vi "SiPM_Oscilloscope_tests.vi"(1 "Results Directory":path=path "C:/Users/johnk/Desktop/ESA_Scintillator_Data", 2 "Isotope":string) -> ()   [LabVIEW 2015]
doc: "This example shows how to configure multiple channels and acquire waveforms from multiple channels."
uses:
  <instrlib>/RIGOL DP800 Series/Public/Channels.ctl
  Agilent_lib/Public/Data/Read Measurement (Current Value).vi
  Agilent_lib/Public/Configure/Trigger/Configure Trigger (Edge).vi
  Agilent_lib/Agilent 2000 3000 X-Series.lvlib
  <vilib>/Analysis/NI_AALPro.lvlib
  <vilib>/Analysis/NI_AALBase.lvlib
  <instrlib>/RIGOL DG4000 Series/RIGOL DG4000 Series.lvlib
  <instrlib>/RIGOL DP800 Series/RIGOL DP800 Series.lvlib
panel:
  in  "x = y?":bool
  in  "Enable\nVernier":bool
  in  "Enable \nREF \nBNC":bool
  in  "Time Base Type":i32(ring) items=["Main", "Window", "XY", "Roll"]
  out "appended array":i32[](array[numeric])
  in  "Tab Control":enum32{"Page 2"}(tab)
  in  "Set Manual Temp?":bool
  in  "Temperature":string
  in  "Settings Button":bool
  in  "Stop Button":bool
  in  "Free Run":bool
  in  "Range":dbl(slide)=0.001 min=2e-08 max=500.0 scale=0.0..0.001
  in  "Pulse Width (s)":ext=1.25e-8 format="%#.3p"
  in  "Read DC":bool
  in  "Out Enable 2":bool
  in  "Set DC":bool
  out "Actual V Level  2":dbl caption="Actual Level (V)" format="%#.3g"
  out "Actual Level (A)":dbl caption="Actual Current Level" format="%#.3g"
  in  "VISA resource name":refnum<visa-resource-name>="USB0::0x0957::0x1780::MY56270584::INSTR"
  out "BIAS Voltage":dbl
  in  "Read Temperature":bool
  out "Celcius":dbl(slide) scale=0.0..30.0
  in  "Trigger Source":i32(ring) items=["Channel 1"=0, "Channel 2"=1, "Channel 3"=2, "Channel 4"=3, "D0"=13, "D1"=14, "D2"=15, "D3"=16, "D4"=17, "D5"=18, "D6"=19, "D7"=20, "D8"=21, "D9"=22, "D10"=23, "D11"=24, "D12"=25, "D13"=26, "D14"=27, "D15"=28, "External"=29, "Power Line"=30, "Waveform Generator"=31]
  in  "Input \nCoupling":i32(ring)=1 items=["AC Coupling", "DC Coupling", "Low Frequency Reject"]
  in  "Edge \nSlope":i32(ring) items=["Pos", "Neg", "Either", "Alt"]
  in  "Trigger Level (V)":dbl(knob)=0.02 min=-10.0 max=10.0 step=0.01 scale=0.0..5.0
  out "HV Indicator":bool
  in  "EN 4":bool
  in  "Ch 4 Vertical Scale":dbl(knob)=5.0 min=0.0 max=5.0 step=0.05 scale=0.0..5.0
  in  "CH 4  offset":dbl(knob) min=-10.0 max=10.0 step=0.01 scale=0.0..10.0
  in  "Ch3 Vertical Scale":dbl(knob)=5.0 min=0.0 max=5.0 step=0.05 scale=0.0..5.0
  in  "CH 3  offset":dbl(knob) min=-10.0 max=10.0 step=0.01 scale=0.0..10.0
  in  "EN 3":bool
  in  "EN 2":bool=TRUE
  in  "Ch 2 Vertical Scale":dbl(knob)=0.05 min=0.0 max=5.0 step=0.05 scale=0.0..5.0
  in  "CH 2  offset":dbl(knob)=0.18 min=-10.0 max=10.0 step=0.01 scale=0.0..10.0
  in  "Ch1 Vertical Scale":dbl(knob)=0.05 min=0.0 max=5.0 step=0.001 scale=0.0..5.0
  in  "CH 1  offset":dbl(knob)=0.18 min=-10.0 max=10.0 step=0.01 scale=0.0..10.0
  in  "EN":bool=TRUE
  out "Oscilloscope Waveform":waveform(dbl)[](graph)
  in  "Impedance":i32(ring)=1 items=["1 MOhm", "50 Ohm"]
  in  "Coupling":i32(ring)=1 items=["AC", "DC"]
  in  "Vertical Setting":i32(ring) items=["Vertical Scale", "Vertical Range"]
  in  "Vertical Range":dbl=40.0
  in  "Time per Division":dbl(knob)=2e-07 scale=0.0..1.0
  in  "Horizontal \nPosition":dbl(knob) scale=0.0..1.0
  in  "Ch1":u8=1 min=1 max=10 step=9
  in  "Ch2":u8=1 min=1 max=10 step=9
  in  "Ch3":u8=10 min=1 max=10 step=9
  in  "Ch4":u8=10 min=1 max=10 step=9
  in  "Start  Auto Tests":bool
  in  "Nb of Steps":u16=20
  out "XY Graph":cluster{dbl[], dbl[]}(graph) caption="Spectrum"
  in  "Step Size (V)":dbl=10.0
  in  "Initial Value (V)":dbl=15.0
  in  "Load file to display":bool
  in  "Select Operation":enum32{"Rec Waveform", "Noise Tests"}(radio)
  in  "VISA session":refnum<visa-resource-name>="USB0::0x1AB1::0x0641::DG4E181901080::INSTR"
  in  "Frequency (Hz)":ext=256000.0 format="%#.3p"
  in  "Amplitude (V)":ext=1.0 format="%.3f"
  in  "Offset (V)":ext=2.3 format="%.3f"
  in  "Output En":bool=TRUE
  in  "Compl":bool
  in  "Set Pulser":bool
  in  "Amplitude Unit":i32(ring) items=["Vpp", "Vrms", "dBm"]
  in  "Z Out (Ohm)":i32=50
  in  "Trigger Mode":i32(ring) items=["Internal", "External", "Manual"]
  in  "Current Limit":dbl=1.0 format="%#.3g"
  in  "Voltage Level":dbl=5.0 caption="Voltage Level (0 V)" format="%#.3g"
  in  "Current Limit 2":dbl=1.0 caption="Current Limit" format="%#.3g"
  in  "Voltage Level 2":dbl=27.3 caption="Voltage Level" format="%#.3g"
  out "Actual Level (V)":dbl caption="Actual Voltage Level" format="%#.3g"
  out "Actual Level (A)":dbl caption="Actual Current Level" format="%#.3g"
  in  "Out Enable":bool
  in  "VISA resource name 2":refnum<visa-resource-name>="USB0::0x1AB1::0x0E11::DP8B181200106::INSTR" caption="VISA resource name"
  out "Frames Recorded":i32
  out "Meas Ind":bool
  in  "Close Session":bool
  in  "File Name":string="1"
  # "NCSR  DEMOKRITOS\nInstitute of Nuclear and Particle Physics\nDetectors Instrumentation Laboratory"
  # "SiPM Scope Tests"
  # "Agilent  DSO-X 6004A Oscilloscope"
  # "KEITHLEY\nElectrometer"
  # "Probe Attenuation"
  # "Record Waveform"
  # "RIGOL DP832A \nDC Power Supply"
  # "RIGOL DG4102 \nFunction Generator"
  # "CH1\n30V/3A"
  # "CH2\n(HV)"
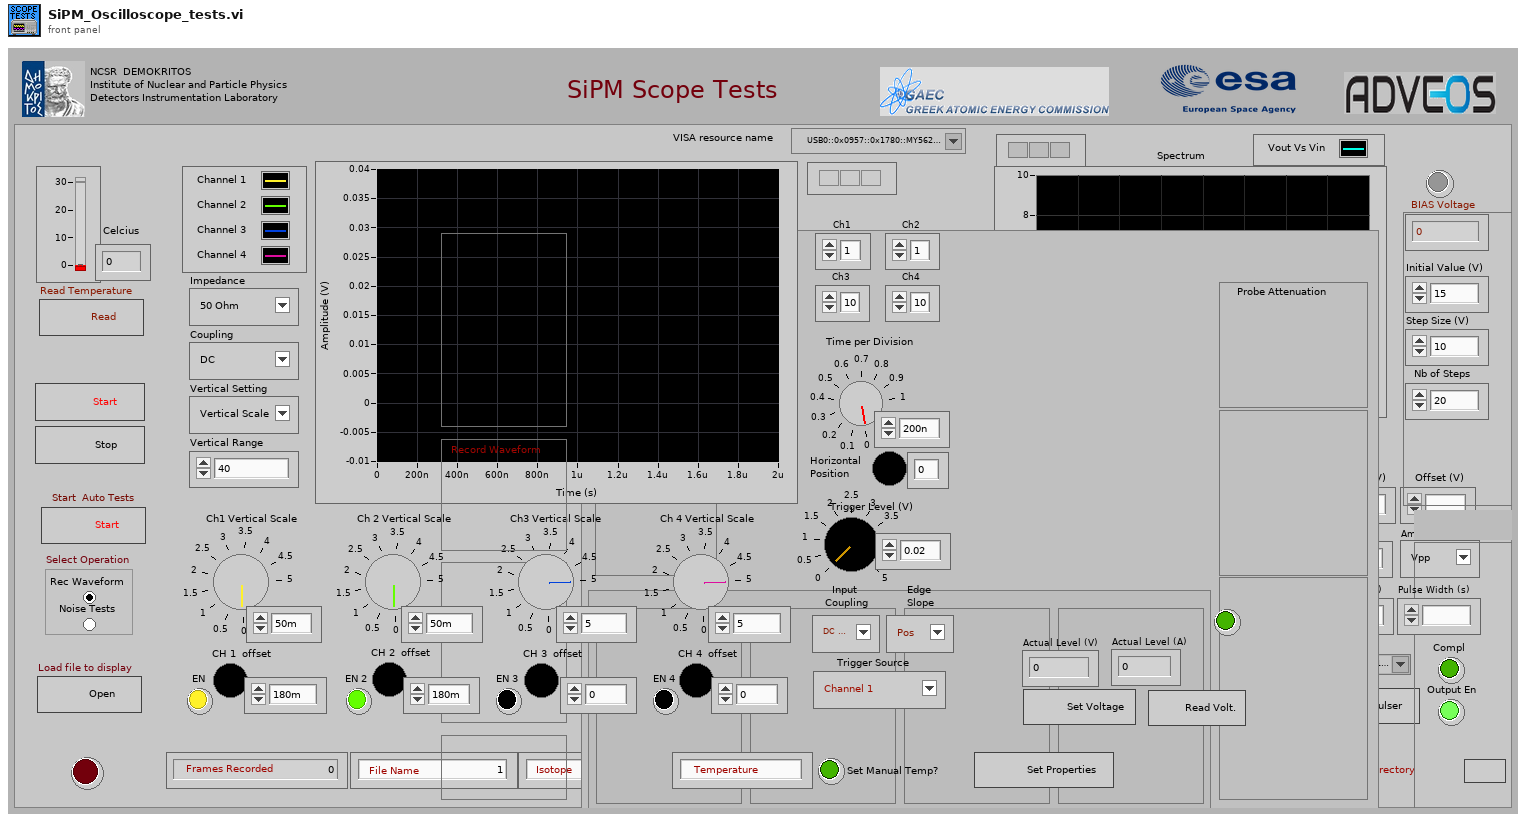
[diagram p1: front panel]
types:
  T1 = enum16{"big-endian, network order", "native, host order", "little-endian"}
  T2 = enum16{"open", "open or create", "create or replace", "create", "open (read-only)"}
  T3 = typedef "RIGOL DP800 Series.lvlib/Channels.ctl" = i32
  T4 = cluster{"X Values":dbl[], "Histogram: h(x)":i32[]}
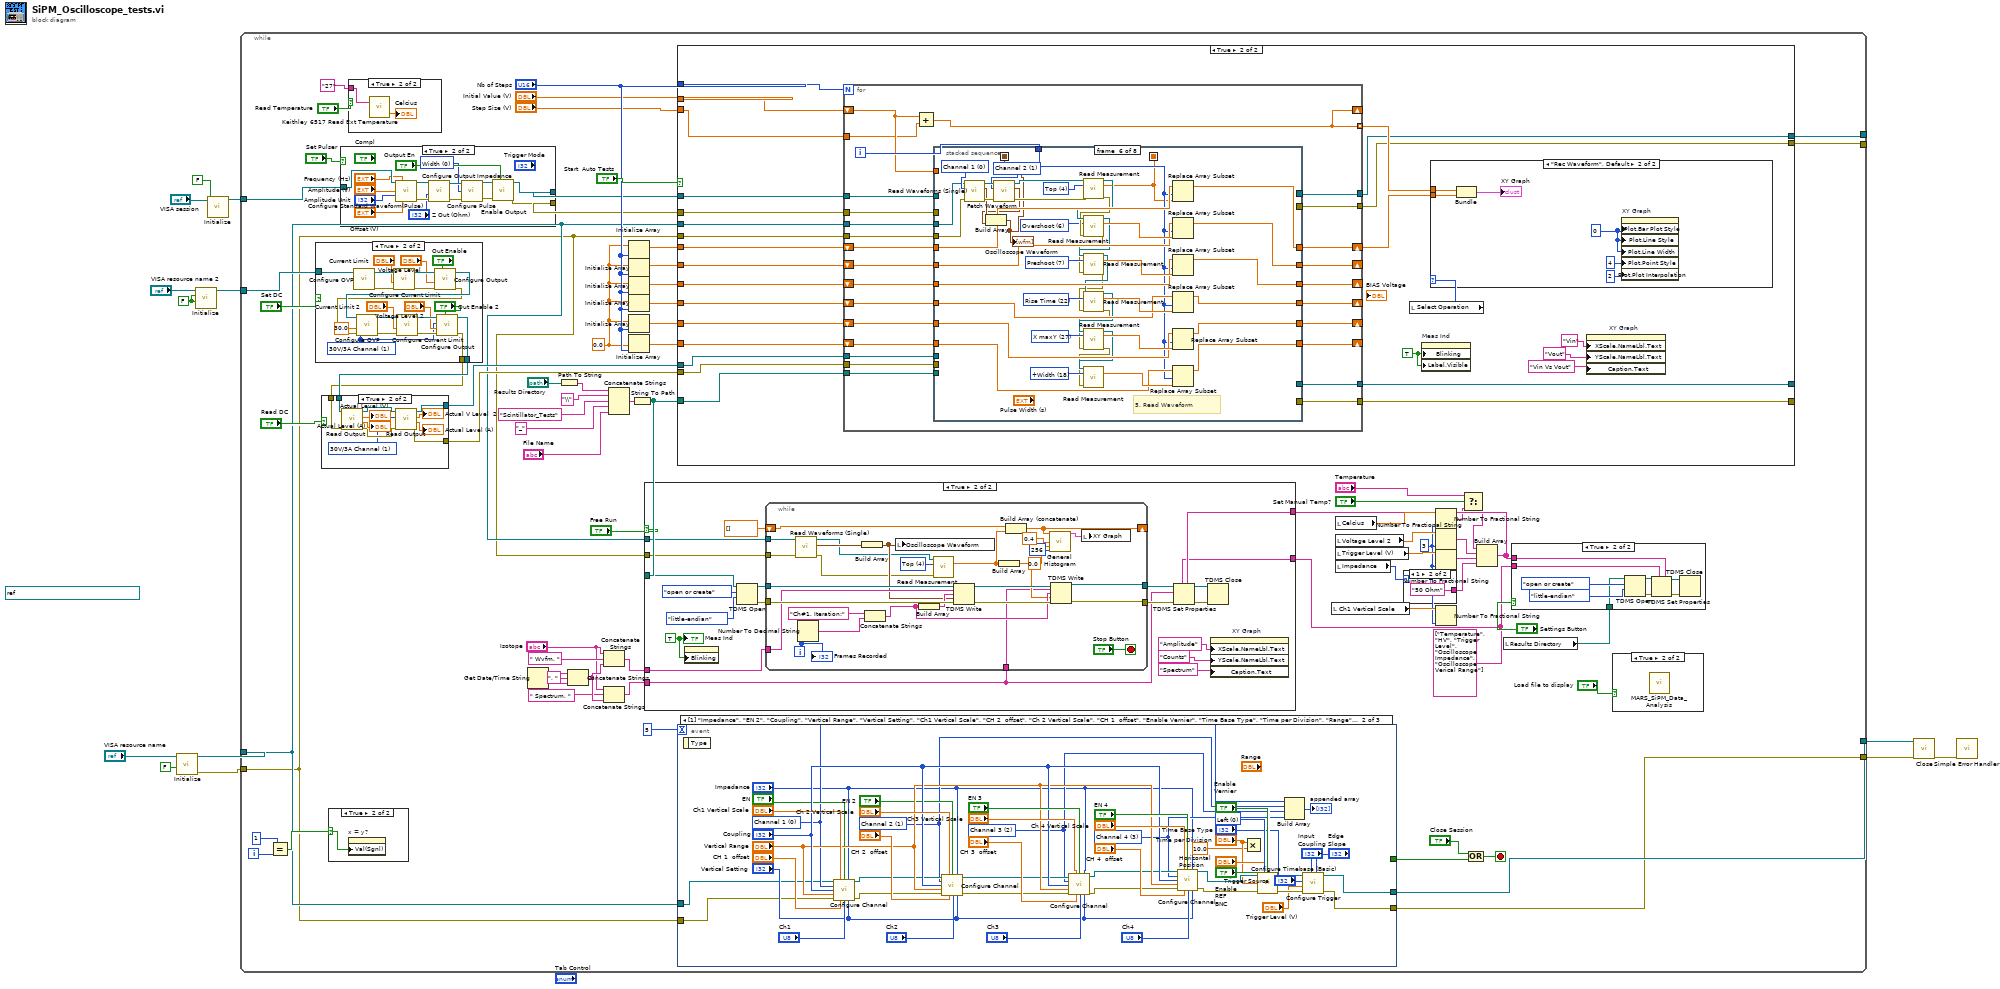
[diagram p0: block diagram]
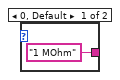
[diagram p2: hidden frame]
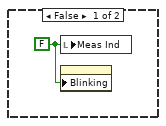
[diagram p4: hidden frame]
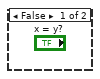
[diagram p7: hidden frame]
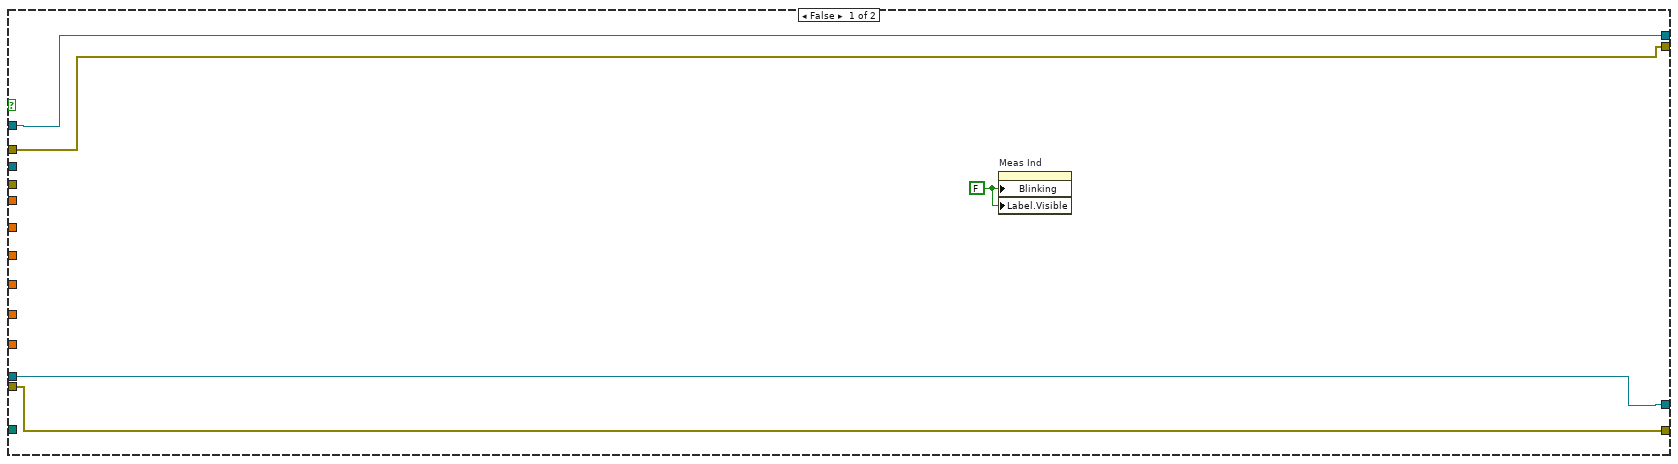
[diagram p11: hidden frame]
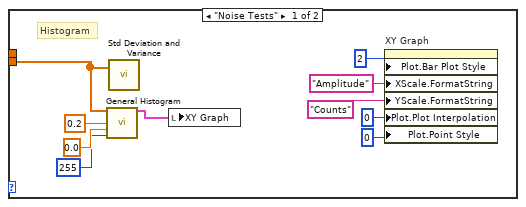
[diagram p12: hidden frame]
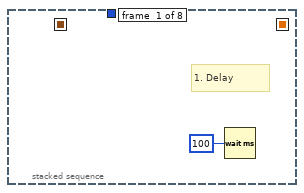
[diagram p13: hidden frame]
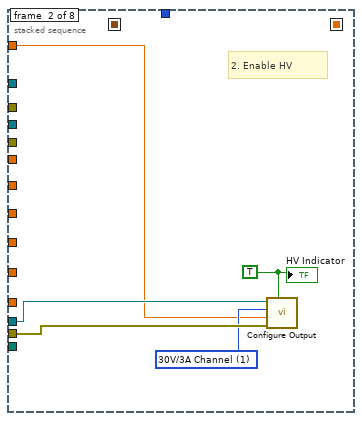
[diagram p14: hidden frame]
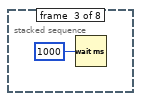
[diagram p15: hidden frame]
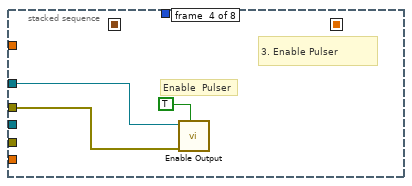
[diagram p16: hidden frame]
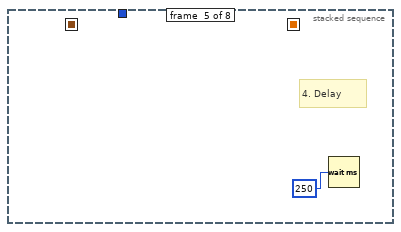
[diagram p17: hidden frame]
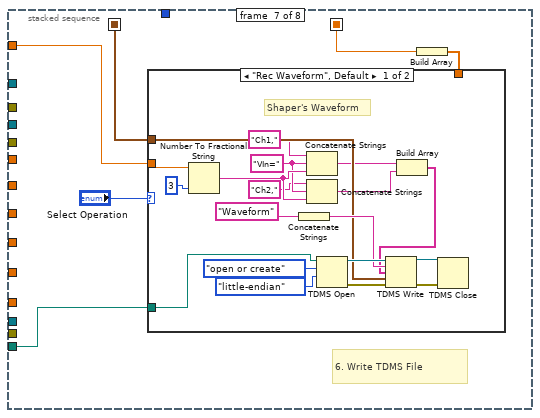
[diagram p18: hidden frame]
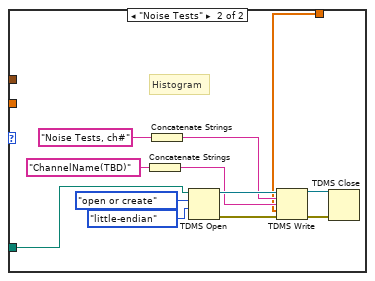
[diagram p19: hidden frame]
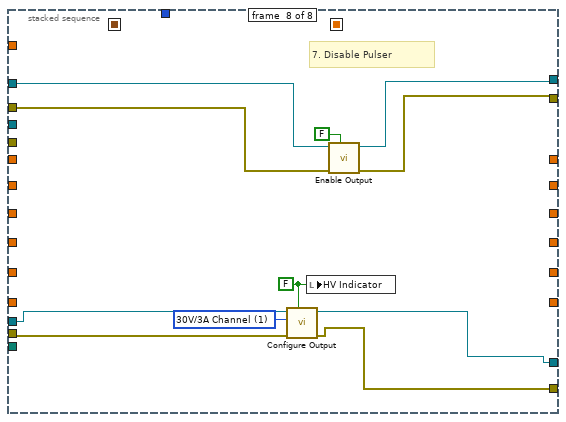
[diagram p20: hidden frame]
diagram:
  w3 = FALSE ("Reset (True)")
  w2 = FALSE ("ID Query (True)")
  (unwired) refnum<visa-resource-name> "USB0::0x0957::0x17A0::MY54100381::INSTR" ("VISA resource name")
  n1 = call <instrlib>:"Initialize.vi"("Reset (True)"=w2, "ID Query (True)"=w2, "VISA resource name"="VISA resource name") -> ("error out"=w11:errorcluster, "VISA resource name out"=w12:refnum<visa-resource-name>)  [unwired: 2 in, 5 out]
  n2 = call <instrlib>:"Initialize.vi"("Reset (True)"=w3, "ID Query (True)"=w3, "VISA resource name"="VISA resource name 2") -> ("VISA resource name out"=w4:refnum<visa-resource-name>)  [unwired: 7 in, 1 out]
  n3 = call <instrlib>:"Initialize.vi"("Reset (True)"=FALSE, "VISA resource name"="VISA session") -> ("VISA resource name out"=w6:refnum<visa-resource-name>)  [unwired: 8 in, 1 out]
  n4 = while {
    tunnel: w12 -> [w44]
    tunnel: w11 -> [w43]
    tunnel: [w76] -> w10
    tunnel: [w75] -> w9
    tunnel: w6 -> [w62]
    tunnel: w4 -> [w54]
    tunnel: [w47] -> _
    tunnel: [w46] -> _
    i -> [w57]
    stop <- w65 stop-if-true
    w18 = string[] ["Temperature", "HV", "Trigger Level", "Oscilloscope Impedance", "Oscilloscope Verical Range"] ("property names")
    w20 = i16 3 ("precision (6)")
    w66 = 0.0 ("element")
    n5 = Equal?(x=1, y=w57) -> (x = y?=w55:bool)
    n6 = case shown="True" "Set DC" {
      tunnel: w54 -> [w161 w180]
      tunnel: [w161 w164] -> w52
      tunnel: [_ w163] -> w51
      frame False {
      }
      frame True {
        w167 = T3 1 items=["30V/3A Channel", "30V/3A Channel", "5V/3A Channel"] ("Channel (0: 30V Channel)")
        n7 = call <instrlib>:"Configure OVP.vi"("VISA resource name"=w180) -> ("error out"=w179:errorcluster, "VISA resource name out"=w182:refnum<visa-resource-name>)  [unwired: 9 in]
        n8 = call <instrlib>:"Configure Current Limit.vi"("error in (no error)"=w179, "Current Limit (5.0 A)"="Current Limit", "VISA resource name"=w182) -> ("error out"=w177:errorcluster, "VISA resource name out"=w181:refnum<visa-resource-name>)  [unwired: 7 in]
        n9 = call <instrlib>:"Configure Output.vi"("Enable Output (T: Enable)"="Out Enable", "error in (no error)"=w177, "Voltage Level (0.0 V)"="Voltage Level", "VISA resource name"=w181) -> ("error out"=w168:errorcluster, "VISA resource name out"=w169:refnum<visa-resource-name>)  [unwired: 6 in]
        n10 = call <instrlib>:"Configure OVP.vi"("error in (no error)"=w168, "Voltage Limit (6.5 V)"=30.0, "Channel (0: 30V Channel)"=w167, "VISA resource name"=w169) -> ("error out"=w173:errorcluster, "VISA resource name out"=w175:refnum<visa-resource-name>)  [unwired: 6 in]
        n11 = call <instrlib>:"Configure Current Limit.vi"("error in (no error)"=w173, "Current Limit (5.0 A)"="Current Limit 2", "VISA resource name"=w175) -> ("error out"=w171:errorcluster, "VISA resource name out"=w174:refnum<visa-resource-name>)  [unwired: 7 in]
        n12 = call <instrlib>:"Configure Output.vi"("Enable Output (T: Enable)"="Out Enable 2", "error in (no error)"=w171, "Voltage Level (0.0 V)"="Voltage Level 2", "Channel (0: 30V Channel)"=w167, "VISA resource name"=w174) -> ("error out"=w163:errorcluster, "VISA resource name out"=w164:refnum<visa-resource-name>)  [unwired: 5 in]
      }
    }
    n13 = case shown="True" "Read DC" {
      tunnel: w52 -> [w149 w154]
      tunnel: w51 -> [w148 w153]
      tunnel: [w149 w151] -> w49
      tunnel: [w148 w150] -> w48
      frame False {
      }
      frame True {
        w152 = T3 1 items=["30V/3A Channel", "30V/3A Channel", "5V/3A Channel"] ("Channel (0: 30V Channel)")
        n14 = call <instrlib>:"Read Output.vi"("error in (no error)"=w153, "VISA resource name"=w154) -> ("error out"=w157:errorcluster, "Actual Current Level (A)"=→"Actual Level (A)":dbl, "Actual Voltage Level (V)"=→"Actual Level (V)":dbl, "VISA resource name out"=w158:refnum<visa-resource-name>)  [unwired: 5 in, 1 out]
        n15 = call <instrlib>:"Read Output.vi"("error in (no error)"=w157, "Channel (0: 30V Channel)"=w152, "VISA resource name"=w158) -> ("error out"=w150:errorcluster, "Actual Current Level (A)"=→"Actual Level (A)":dbl, "Actual Voltage Level (V)"=→"Actual V Level  2":dbl, "VISA resource name out"=w151:refnum<visa-resource-name>)  [unwired: 4 in, 1 out]
      }
    }
    n16 = case shown="True" w55 {
      selector: w55 -> [_ w183]
      frame False {
      }
      frame True {
        n17 = property on="x = y?" class="Bool (strict)"("Val(Sgnl)"=w183) -> ()  [unwired: 2 in, 2 out]
      }
    }
    n18 = case shown="True" "Set Pulser" {
      tunnel: w62 -> [w186 w202]
      tunnel: [w186 w196] -> w45
      tunnel: [_ w197] -> w60
      frame False {
      }
      frame True {
        w187 = 0 items=["Width", "Duty"] ("Pulse Hold (1: Duty)")
        n19 = call <instrlib>:"Configure Standard Waveform(Pulse).vi"("VISA resource name"=w202, "Frequency (1000 Hz)"="Frequency (Hz)", "Amplitude (5)"="Amplitude (V)", "Amplitude Unit (0: Vpp)"="Amplitude Unit", "Offset (0)"="Offset (V)") -> ("VISA resource name out"=w194:refnum<visa-resource-name>, "error out"=w193:errorcluster)  [unwired: 9 in]
        n20 = call <instrlib>:"Configure Output Impedance.vi"("error in (no error)"=w193, "Output Impedance (50 Ohm)"="Z Out (Ohm)", "VISA resource name"=w194) -> ("error out"=w190:errorcluster, "VISA resource name out"=w191:refnum<visa-resource-name>)  [unwired: 7 in]
        n21 = call "Configure Pulse.vi"("VISA resource name"=w191, "Pulse Hold (1: Duty)"=w187, "error in (no error)"=w190) -> ("VISA resource name out"=w189:refnum<visa-resource-name>, "error out"=w188:errorcluster)  [unwired: 11 in]
        n22 = call "Enable Output.vi"("Enable Output (T: Enable)"="Output En", "error in (no error)"=w188, "VISA resource name"=w189) -> ("error out"=w197:errorcluster, "VISA resource name out"=w196:refnum<visa-resource-name>)  [unwired: 7 in]
      }
    }
    n23 = case shown="True" "Read Temperature" {
      tunnel: "27" ("GPIB address") -> [_ w185]
      frame False {
      }
      frame True {
        n24 = call "Keithley 6517 Read Ext Temperature.vi"("GPIB address"=w185) -> ("External Temperature"=→"Celcius":dbl)  [unwired: 1 in, 1 out]
      }
    }
    n25 = Get Date/Time String() -> (date string=w37:string, time string=w39:string)  [unwired: 3 in]
    n26 = Path To String(path="Results Directory") -> (string=w71:string)
    n27 = Concatenate Strings(w37, ", " ("string"), w39) -> (w38:string)
    n28 = Concatenate Strings("Isotope", " Wvfm, " ("group name in (Untitled)"), w38) -> (w32:string)
    n29 = Concatenate Strings("Isotope", " Spectrum, " ("group name in (Untitled)"), w38) -> (w31:string)
    n30 = Concatenate Strings(w71, "\\" ("string"), "Scintillator_Tests", "_", "File Name") -> (w69:string)
    n31 = Initialize Array(w66, "Nb of Steps") -> (w85:dbl[])
    n32 = Initialize Array(w66, "Nb of Steps") -> (w82:dbl[])
    n33 = Initialize Array(w66, "Nb of Steps") -> (w81:dbl[])
    n34 = Initialize Array(w66, "Nb of Steps") -> (w80:dbl[])
    n35 = Initialize Array(w66, "Nb of Steps") -> (w79:dbl[])
    n36 = Initialize Array(w66, "Nb of Steps") -> (w77:dbl[])
    n37 = String To Path(string=w69) -> (path=w42:path)
    n38 = case shown="True" "Start  Auto Tests" {
      tunnel: w44 -> [_ w234]
      tunnel: w43 -> [_ w233]
      tunnel: "Nb of Steps" -> [_ w232]
      tunnel: "Step Size (V)" -> [_ w217]
      tunnel: "Initial Value (V)" -> [_ w218]
      tunnel: w85 -> [_ w231]
      tunnel: w45 -> [w204 w220]
      tunnel: w82 -> [_ w230]
      tunnel: w81 -> [_ w229]
      tunnel: w80 -> [_ w228]
      tunnel: w79 -> [_ w227]
      tunnel: w77 -> [_ w226]
      tunnel: w42 -> [_ w222]
      tunnel: w60 -> [w203 w219]
      tunnel: w49 -> [w206 w216]
      tunnel: w48 -> [w205 w215]
      tunnel: [w206 w214] -> _
      tunnel: [w205 w213] -> _
      tunnel: [w204 w212] -> w47
      tunnel: [w203 w211] -> w46
      frame False {
        w207 = FALSE ("Blinking")
        n39 = property on="Meas Ind" class="Bool (strict)"("Blinking"=w207, "Label.Visible"=w207) -> ()  [unwired: 2 in, 2 out]
      }
      frame True {
        w221 = TRUE ("Blinking")
        n40 = for {
          N: w232 -> [_]
          tunnel: w234 -> [w274]
          tunnel: w233 -> [w273]
          shift-right: [w271] -> w223
          shift-left: w231 -> [w272]
          tunnel: [w258] -> w224 mode=indexing
          tunnel: w217 -> [w257]
          tunnel: w220 -> [w276]
          tunnel: w219 -> [w275]
          shift-right: [w269] -> _
          shift-left: w230 -> [w270]
          shift-right: [w267] -> _
          shift-left: w229 -> [w268]
          shift-right: [w265] -> _
          shift-left: w228 -> [w266]
          shift-right: [w263] -> _
          shift-left: w227 -> [w264]
          shift-right: [w261] -> _
          shift-left: w226 -> [w262]
          tunnel: w222 -> [w260]
          shift-right: [w258] -> _
          shift-left: w218 -> [w259]
          tunnel: w216 -> [w256]
          tunnel: w215 -> [w255]
          tunnel: [w254] -> w214
          tunnel: [w253] -> w213
          tunnel: [w252] -> w212
          tunnel: [w251] -> w211
          i -> [w277]
          n41 = Add(x=w259, y=w257) -> (x+y=w258:dbl)
          n42 = stacked-sequence {
            seq-local: [_ _ _ _ _ w289 _ _] -> [_ _ _ _ _ _ w340 _]
            seq-local: [_ _ _ _ _ w297 _ _] -> [_ _ _ _ _ _ w338 _]
            tunnel: w259 -> [_ w280 _ _ _ _ w335 _]
            tunnel: w277 -> [_ _ _ _ _ w300 _ _]
            tunnel: w276 -> [_ _ _ w287 _ _ _ w382]
            tunnel: w275 -> [_ _ _ w286 _ _ _ w381]
            tunnel: w274 -> [_ _ _ _ _ w332 _ _]
            tunnel: w273 -> [_ _ _ _ _ w331 _ _]
            tunnel: w272 -> [_ _ _ _ _ w330 _ _]
            tunnel: [_ _ _ _ _ w298 _ _] -> w271
            tunnel: w270 -> [_ _ _ _ _ w325 _ _]
            tunnel: [_ _ _ _ _ w324 _ _] -> w269
            tunnel: w268 -> [_ _ _ _ _ w319 _ _]
            tunnel: [_ _ _ _ _ w318 _ _] -> w267
            tunnel: w266 -> [_ _ _ _ _ w313 _ _]
            tunnel: [_ _ _ _ _ w312 _ _] -> w265
            tunnel: w264 -> [_ _ _ _ _ w309 _ _]
            tunnel: [_ _ _ _ _ w306 _ _] -> w263
            tunnel: w262 -> [_ _ _ _ _ w303 _ _]
            tunnel: [_ _ _ _ _ w299 _ _] -> w261
            tunnel: w260 -> [_ _ _ _ _ _ w336 _]
            tunnel: w256 -> [_ w283 _ _ _ _ _ w377]
            tunnel: w255 -> [_ w282 _ _ _ _ _ w376]
            tunnel: [_ _ _ _ _ _ _ w373] -> w254
            tunnel: [_ _ _ _ _ _ _ w372] -> w253
            tunnel: [_ _ _ _ _ _ _ w379] -> w252
            tunnel: [_ _ _ _ _ _ _ w378] -> w251
            frame #0 {
              # "1. Delay"
              n43 = Wait (ms)(milliseconds to wait=u32 100) -> ()  [unwired: 1 out]
            }
            frame #1 {
              w281 = T3 1 items=["30V/3A Channel", "30V/3A Channel", "5V/3A Channel"] ("Channel (0: 30V Channel)")
              w279 = TRUE ("V-Source Operate")
              # "2. Enable HV"
              n44 = call <instrlib>:"Configure Output.vi"("Enable Output (T: Enable)"=w279, "error in (no error)"=w282, "Voltage Level (0.0 V)"=w280, "Channel (0: 30V Channel)"=w281, "VISA resource name"=w283) -> ()  [unwired: 5 in, 2 out]
              "HV Indicator" <- w279
            }
            frame #2 {
              n45 = Wait (ms)(milliseconds to wait=u32 1000) -> ()  [unwired: 1 out]
            }
            frame #3 {
              # "3. Enable Pulser"
              # "Enable  Pulser"
              n46 = call "Enable Output.vi"("Enable Output (T: Enable)"=TRUE, "error in (no error)"=w286, "VISA resource name"=w287) -> ()  [unwired: 7 in, 2 out]
            }
            frame #4 {
              # "4. Delay"
              n47 = Wait (ms)(milliseconds to wait=u32 250 ("Delay (ms)")) -> ()  [unwired: 1 out]
            }
            frame #5 {
              w292 = 1 items=["Channel 1"=0, "Channel 2"=1, "Channel 3"=2, "Channel 4"=3, "Waveform Memory 1"=5, "Waveform Memory 2"=6, "Serial Bus 1"=7, "Serial Bus 2"=8, "Digital Bus Low"=9, "Digital Bus High "=10, "Digital Bus 1"=11, "Digital Bus 2"=12, "Function 1"=32, "Function 2"=33, "Function 3"=34, "Function 4"=35, "Math 1"=36, "Math 2"=37, "Math 3"=38, "Math 4"=39] ("Source Channel (0: Channel 1)")
              w305 = 18 items=["Peak-Peak", "Maximum", "Mimimum", "Amplitude", "Top", "Base", "Overshoot", "Preshoot", "Average - N Cycles", "Average - Full Screen", "DC RMS - N Cycles", "DC RMS - Full Screen", "AC RMS - N Cycles", "AC RMS - Full Screen (Std Dev)", "Ratio", "Period", "Frequency", "Counter", "+Width", "-Width", "Burst Width", "Duty Cycle", "Rise Time", "Fall Time", "Delay", "Phase", "X minY", "X maxY", "Positive Pulse Count", "Negative Pulse Count", "Raising Edge Count", "Falling Edge Count", "Area - N Cycle", "Area - Full Screen", "Nth Edge Time", "Nth Edge Cross Level Time"] ("Measurement Type (0: Peak-Peak)")
              w311 = 27 items=["Peak-Peak", "Maximum", "Mimimum", "Amplitude", "Top", "Base", "Overshoot", "Preshoot", "Average - N Cycles", "Average - Full Screen", "DC RMS - N Cycles", "DC RMS - Full Screen", "AC RMS - N Cycles", "AC RMS - Full Screen (Std Dev)", "Ratio", "Period", "Frequency", "Counter", "+Width", "-Width", "Burst Width", "Duty Cycle", "Rise Time", "Fall Time", "Delay", "Phase", "X minY", "X maxY", "Positive Pulse Count", "Negative Pulse Count", "Raising Edge Count", "Falling Edge Count", "Area - N Cycle", "Area - Full Screen", "Nth Edge Time", "Nth Edge Cross Level Time"] ("Measurement Type (0: Peak-Peak)")
              w317 = 22 items=["Peak-Peak", "Maximum", "Mimimum", "Amplitude", "Top", "Base", "Overshoot", "Preshoot", "Average - N Cycles", "Average - Full Screen", "DC RMS - N Cycles", "DC RMS - Full Screen", "AC RMS - N Cycles", "AC RMS - Full Screen (Std Dev)", "Ratio", "Period", "Frequency", "Counter", "+Width", "-Width", "Burst Width", "Duty Cycle", "Rise Time", "Fall Time", "Delay", "Phase", "X minY", "X maxY", "Positive Pulse Count", "Negative Pulse Count", "Raising Edge Count", "Falling Edge Count", "Area - N Cycle", "Area - Full Screen", "Nth Edge Time", "Nth Edge Cross Level Time"] ("Measurement Type (0: Peak-Peak)")
              w323 = 7 items=["Peak-Peak", "Maximum", "Mimimum", "Amplitude", "Top", "Base", "Overshoot", "Preshoot", "Average - N Cycles", "Average - Full Screen", "DC RMS - N Cycles", "DC RMS - Full Screen", "AC RMS - N Cycles", "AC RMS - Full Screen (Std Dev)", "Ratio", "Period", "Frequency", "Counter", "+Width", "-Width", "Burst Width", "Duty Cycle", "Rise Time", "Fall Time", "Delay", "Phase", "X minY", "X maxY", "Positive Pulse Count", "Negative Pulse Count", "Raising Edge Count", "Falling Edge Count", "Area - N Cycle", "Area - Full Screen", "Nth Edge Time", "Nth Edge Cross Level Time"] ("Measurement Type (0: Peak-Peak)")
              w327 = 6 items=["Peak-Peak", "Maximum", "Mimimum", "Amplitude", "Top", "Base", "Overshoot", "Preshoot", "Average - N Cycles", "Average - Full Screen", "DC RMS - N Cycles", "DC RMS - Full Screen", "AC RMS - N Cycles", "AC RMS - Full Screen (Std Dev)", "Ratio", "Period", "Frequency", "Counter", "+Width", "-Width", "Burst Width", "Duty Cycle", "Rise Time", "Fall Time", "Delay", "Phase", "X minY", "X maxY", "Positive Pulse Count", "Negative Pulse Count", "Raising Edge Count", "Falling Edge Count", "Area - N Cycle", "Area - Full Screen", "Nth Edge Time", "Nth Edge Cross Level Time"] ("Measurement Type (0: Peak-Peak)")
              w333 = 4 items=["Peak-Peak", "Maximum", "Mimimum", "Amplitude", "Top", "Base", "Overshoot", "Preshoot", "Average - N Cycles", "Average - Full Screen", "DC RMS - N Cycles", "DC RMS - Full Screen", "AC RMS - N Cycles", "AC RMS - Full Screen (Std Dev)", "Ratio", "Period", "Frequency", "Counter", "+Width", "-Width", "Burst Width", "Duty Cycle", "Rise Time", "Fall Time", "Delay", "Phase", "X minY", "X maxY", "Positive Pulse Count", "Negative Pulse Count", "Raising Edge Count", "Falling Edge Count", "Area - N Cycle", "Area - Full Screen", "Nth Edge Time", "Nth Edge Cross Level Time"] ("Measurement Type (0: Peak-Peak)")
              w334 = 0 items=["Channel 1"=0, "Channel 2"=1, "Channel 3"=2, "Channel 4"=3, "Waveform Memory 1"=5, "Waveform Memory 2"=6, "Serial Bus 1"=7, "Serial Bus 2"=8, "Digital Bus Low"=9, "Digital Bus High "=10, "Digital Bus 1"=11, "Digital Bus 2"=12, "Function 1"=32, "Function 2"=33, "Function 3"=34, "Function 4"=35, "Math 1"=36, "Math 2"=37, "Math 3"=38, "Math 4"=39] ("Source Channel (0: Channel 1)")
              # "5. Read Waveform"
              n48 = call "Read Waveforms (Single).vi"("error in (no error)"=w331, "Source Channel (0: Channel 1)"=w334, "VISA resource name"=w332) -> ("error out"=w294:errorcluster, "Waveform Data"=w291:waveform(dbl), "VISA resource name out"=w296:refnum<visa-resource-name>)  [unwired: 6 in]
              n49 = call "Fetch Waveform.vi"("error in (no error)"=w294, "Source Channel (0: Channel 1)"=w292, "VISA resource name"=w296) -> ("error out"=w293:errorcluster, "Waveform Data"=w290:waveform(dbl), "VISA resource name out"=w295:refnum<visa-resource-name>)  [unwired: 6 in]
              n50 = Build Array(w291, w290) -> (w289:waveform(dbl)[])
              "Oscilloscope Waveform" <- w289
              n51 = call-poly "Read Measurement.vi"("VISA resource name"=w295, "Measurement Type (0: Peak-Peak)"=w333, "error in (no error)"=w293) -> ("VISA resource name out"=w329:refnum<visa-resource-name>, "Result Value"=w297:dbl, "error out"=w328:errorcluster)  [unwired: 10 in]
              n52 = call-poly "Read Measurement.vi"("VISA resource name"=w329, "Measurement Type (0: Peak-Peak)"=w327, "error in (no error)"=w328) -> ("VISA resource name out"=w321:refnum<visa-resource-name>, "Result Value"=w326:dbl, "error out"=w320:errorcluster)  [unwired: 10 in]
              n53 = call-poly "Read Measurement.vi"("VISA resource name"=w321, "Measurement Type (0: Peak-Peak)"=w323, "error in (no error)"=w320) -> ("VISA resource name out"=w316:refnum<visa-resource-name>, "Result Value"=w322:dbl, "error out"=w315:errorcluster)  [unwired: 10 in]
              n54 = call-poly "Read Measurement.vi"("VISA resource name"=w316, "Measurement Type (0: Peak-Peak)"=w317, "error in (no error)"=w315) -> ("VISA resource name out"=w308:refnum<visa-resource-name>, "Result Value"=w314:dbl, "error out"=w307:errorcluster)  [unwired: 10 in]
              n55 = call-poly "Read Measurement.vi"("VISA resource name"=w308, "Measurement Type (0: Peak-Peak)"=w311, "error in (no error)"=w307) -> ("VISA resource name out"=w302:refnum<visa-resource-name>, "Result Value"=w310:dbl, "error out"=w301:errorcluster)  [unwired: 10 in]
              n56 = call-poly "Read Measurement.vi"("VISA resource name"=w302, "Measurement Type (0: Peak-Peak)"=w305, "error in (no error)"=w301) -> ("Result Value"=w304:dbl)  [unwired: 10 in, 2 out]
              n57 = Replace Array Subset(array=w330, new element=w297, index=w300) -> (w298:dbl[])
              n58 = Replace Array Subset(array=w325, new element=w326, index=w300) -> (w324:dbl[])
              n59 = Replace Array Subset(array=w319, new element=w322, index=w300) -> (w318:dbl[])
              n60 = Replace Array Subset(array=w313, new element=w314, index=w300) -> (w312:dbl[])
              n61 = Replace Array Subset(array=w309, new element=w310, index=w300) -> (w306:dbl[])
              n62 = Replace Array Subset(array=w303, new element=w304, index=w300) -> (w299:dbl[])
            }
            frame #6 {
              # "6. Write TDMS File"
              n63 = Build Array(w338) -> (w339:dbl[])
              n64 = case shown="\"Rec Waveform\", Default" "Select Operation" {
                tunnel: w340 -> [w351 _]
                tunnel: w339 -> [_ w362]
                tunnel: w336 -> [w350 w361]
                tunnel: w335 -> [w347 _]
                frame "Rec Waveform", Default {
                  w343 = "VIn=" ("group name in (Untitled)")
                  # "Shaper's Waveform"
                  n65 = Number To Fractional String(number=w347, precision (6)=i16 3) -> (F-format string=w344:string)  [unwired: 2 in]
                  n66 = Concatenate Strings("Waveform" ("group name in (Untitled)")) -> (w352:string)
                  n67 = Concatenate Strings("Ch1," ("string"), w343, w344) -> (w349:string)
                  n68 = Concatenate Strings("Ch2," ("string"), w343, w344) -> (w341:string)
                  n69 = TDMS Open(9:T1."little-endian" ("byte order (2:little-endian)"), 10:T2."open or create" ("operation (0:open)"), 11:w350) -> (0:w356:errorcluster, 3:w359:refnum<k34>)  [unwired: 4 in]
                  n70 = Build Array(w349, w341) -> (w348:string[])
                  n71 = TDMS Write(0:w359, 5:w352, 7:w348, 9:w351, 11:w356) -> (4:w354:refnum<k34>, 15:w355:errorcluster)  [unwired: 1 in, 2 out]
                  n72 = TDMS Close(8:w355, 11:w354) -> ()  [unwired: 2 out]
                }
                frame "Noise Tests" {
                  # "Histogram"
                  n73 = Concatenate Strings("ChannelName(TBD)" ("string")) -> (w363:string)
                  n74 = Concatenate Strings("Noise Tests, ch#" ("group name in (Untitled)")) -> (w364:string)
                  n75 = TDMS Open(9:T1."little-endian" ("byte order (2:little-endian)"), 10:T2."open or create" ("operation (0:open)"), 11:w361) -> (0:w368:errorcluster, 3:w371:refnum<k34>)  [unwired: 4 in]
                  n76 = TDMS Write(0:w371, 5:w364, 7:w363, 9:w362, 11:w368) -> (4:w366:refnum<k34>, 15:w367:errorcluster)  [unwired: 1 in, 2 out]
                  n77 = TDMS Close(8:w367, 11:w366) -> ()  [unwired: 2 out]
                }
              }
            }
            frame #7 {
              w375 = T3 1 items=["30V/3A Channel", "30V/3A Channel", "5V/3A Channel"] ("Channel (0: 30V Channel)")
              w374 = FALSE ("V-Source Operate")
              # "7. Disable Pulser"
              n78 = call <instrlib>:"Configure Output.vi"("Enable Output (T: Enable)"=w374, "error in (no error)"=w376, "Channel (0: 30V Channel)"=w375, "VISA resource name"=w377) -> ("error out"=w372:errorcluster, "VISA resource name out"=w373:refnum<visa-resource-name>)  [unwired: 6 in]
              n79 = local write "HV Indicator"(w374) -> ()
              n80 = call "Enable Output.vi"("Enable Output (T: Enable)"=FALSE, "error in (no error)"=w381, "VISA resource name"=w382) -> ("error out"=w378:errorcluster, "VISA resource name out"=w379:refnum<visa-resource-name>)  [unwired: 7 in]
            }
          }
        }
        n81 = local read "Select Operation"() -> (w225:enum32{"Rec Waveform", "Noise Tests"})
        n82 = property on="Meas Ind" class="Bool (strict)"("Blinking"=w221, "Label.Visible"=w221) -> ()  [unwired: 2 in, 2 out]
        n83 = case shown="\"Rec Waveform\", Default" w225 {
          tunnel: w224 -> [_ w250]
          tunnel: w223 -> [w236 w249]
          frame "Noise Tests" {
            # "Histogram"
            n84 = call <vilib>:"General Histogram.vi"("X"=w236, "max"=0.2, "min"=0.0, "# bins"=255) -> ("Histogram Graph"=w241:T4)  [unwired: 7 in, 4 out]
            n85 = call <vilib>:"Std Deviation and Variance.vi"("X"=w236) -> ()  [unwired: 1 in, 3 out]
            n86 = local write "XY Graph"(w241) -> ()
            n87 = property on="XY Graph" class="XYGraph (strict)"("Plot.Bar Plot Style"=u8 2, "XScale.FormatString"="Amplitude" ("X Scale.Format String"), "YScale.FormatString"="Counts" ("Y Scale.Format String"), "Plot.Plot Interpolation"=u8 0, "Plot.Point Style"=u8 0) -> ()  [unwired: 2 in, 2 out]
          }
          frame "Rec Waveform", Default {
            w248 = u8 0 ("Plot.Bar Plot Style")
            n88 = Bundle(w250, w249) -> (→"XY Graph":cluster{dbl[], dbl[]})  [unwired: 1 in]
            n89 = property on="XY Graph" class="XYGraph (strict)"("Plot.Bar Plot Style"=w248, "Plot.Line Style"=w248, "Plot.Line Width"=w248, "Plot.Point Style"=u8 4, "Plot.Plot Interpolation"=u8 2) -> ()  [unwired: 2 in, 2 out]
          }
        }
        n90 = property on="XY Graph" class="XYGraph (strict)"("XScale.NameLbl.Text"="Vin" ("X Scale.Unit Label.Text"), "YScale.NameLbl.Text"="Vout" ("Y Scale.Name Label.Text"), "Caption.Text"="Vin Vs Vout") -> ()  [unwired: 2 in, 2 out]
      }
    }
    n91 = event shown="[1] \"Impedance\", \"EN 2\", \"Coupling\", \"Vertical Range\", \"Vertical Setting\", \"Ch1 Vertical Scale\", \"CH 2  offset\", \"Ch 2 Vertical Scale\", \"CH 1  offset\", \"Enable Vernier\", \"Time Base Type\", \"Time per Division\", \"Range\", \"Horizontal  Position\", \"Enable  REF  BNC\", \"EN\", \"EN 3\", \"CH 4  offset\", \"CH 3  offset\", \"Ch 4 Vertical Scale\", \"EN 4\", \"Ch3 Vertical Scale\", \"Trigger Level (V)\", \"Input  Coupling\", \"x = y?\": Value Change" {
      selector: _ -> [_ _ _]
      dyn-events: _ -> [_ _ _]
      timeout: 5 -> [_ _ _]
      tunnel: w44 -> [w384 w398 _]
      tunnel: w43 -> [w383 w397 _]
      tunnel: [w384 w394 _] -> w76
      tunnel: [w383 w392 _] -> w75
      tunnel: [_ _ TRUE ("y")] -> w63
      event Timeout {
        n92 = event-data() -> ()  [unwired: 1 in, 2 out]
      }
      event "Impedance", "EN 2", "Coupling", "Vertical Range", "Vertical Setting", "Ch1 Vertical Scale", "CH 2  offset", "Ch 2 Vertical Scale", "CH 1  offset", "Enable\nVernier", "Time Base Type", "Time per Division", "Range", "Horizontal \nPosition", "Enable \nREF \nBNC", "EN", "EN 3", "CH 4  offset", "CH 3  offset", "Ch 4 Vertical Scale", "EN 4", "Ch3 Vertical Scale", "Trigger Level (V)", "Input \nCoupling", "x = y?": Value Change {
        w426 = 0 items=["Left", "Center", "Right"] ("Reference")
        w399 = 3 items=["Channel 1", "Channel 2", "Channel 3", "Channel 4"] ("Channel Name (0: Channel 1)")
        w400 = 2 items=["Channel 1", "Channel 2", "Channel 3", "Channel 4"] ("Channel Name (0: Channel 1)")
        w401 = 1 items=["Channel 1", "Channel 2", "Channel 3", "Channel 4"] ("Channel Name (0: Channel 1)")
        w402 = 0 items=["Channel 1", "Channel 2", "Channel 3", "Channel 4"] ("Channel Name (0: Channel 1)")
        n93 = event-data() -> ()  [unwired: 1 in, 1 out]
        n94 = call "Configure Channel.vi"("VISA resource name"=w398, "Vertical Scale (5.0 V)"="Ch1 Vertical Scale", "Enable Channel (T: Enable)"="EN", "Impedance (0: 1 MOhm)"="Impedance", "Channel Name (0: Channel 1)"=w402, "Coupling (1: DC)"="Coupling", "Vertical Range (40.0 V)"="Vertical Range", "error in (no error)"=w397, "Vertical Offset (0.0)"="CH 1  offset", "Probe Attenuation (1.0)"="Ch1", "Vertical Setting (1: Vertical Range)"="Vertical Setting") -> ("VISA resource name out"=w412:refnum<visa-resource-name>, "error out"=w411:errorcluster)  [unwired: 3 out]
        n95 = call "Configure Channel.vi"("VISA resource name"=w412, "Vertical Scale (5.0 V)"="Ch 2 Vertical Scale", "Enable Channel (T: Enable)"="EN 2", "Impedance (0: 1 MOhm)"="Impedance", "Channel Name (0: Channel 1)"=w401, "Coupling (1: DC)"="Coupling", "Vertical Range (40.0 V)"="Vertical Range", "error in (no error)"=w411, "Vertical Offset (0.0)"="CH 2  offset", "Probe Attenuation (1.0)"="Ch2", "Vertical Setting (1: Vertical Range)"="Vertical Setting") -> ("VISA resource name out"=w410:refnum<visa-resource-name>, "error out"=w409:errorcluster)  [unwired: 3 out]
        n96 = call "Configure Channel.vi"("VISA resource name"=w410, "Vertical Scale (5.0 V)"="Ch3 Vertical Scale", "Enable Channel (T: Enable)"="EN 3", "Impedance (0: 1 MOhm)"="Impedance", "Channel Name (0: Channel 1)"=w400, "Coupling (1: DC)"="Coupling", "Vertical Range (40.0 V)"="Vertical Range", "error in (no error)"=w409, "Vertical Offset (0.0)"="CH 3  offset", "Probe Attenuation (1.0)"="Ch3", "Vertical Setting (1: Vertical Range)"="Vertical Setting") -> ("VISA resource name out"=w408:refnum<visa-resource-name>, "error out"=w407:errorcluster)  [unwired: 3 out]
        n97 = call "Configure Channel.vi"("VISA resource name"=w408, "Vertical Scale (5.0 V)"="Ch 4 Vertical Scale", "Enable Channel (T: Enable)"="EN 4", "Impedance (0: 1 MOhm)"="Impedance", "Channel Name (0: Channel 1)"=w399, "Coupling (1: DC)"="Coupling", "Vertical Range (40.0 V)"="Vertical Range", "error in (no error)"=w407, "Vertical Offset (0.0)"="CH 4  offset", "Probe Attenuation (1.0)"="Ch4", "Vertical Setting (1: Vertical Range)"="Vertical Setting") -> ("VISA resource name out"=w406:refnum<visa-resource-name>, "error out"=w405:errorcluster)  [unwired: 3 out]
        n98 = Multiply(x="Time per Division", y=10.0) -> ()  [unwired: 1 out]
        n99 = call "Configure Timebase (Basic).vi"("VISA resource name"=w406, "Reference (1: Center)"=w426, "Enable Vernier (F: Disable)"="Enable\nVernier", "Time Base Type (0: Main)"="Time Base Type", "Scale (50 s/div)"="Time per Division", "error in (no error)"=w405, "Position (0.0)"="Horizontal \nPosition", "Enable REF BNC (F: Disable)"="Enable \nREF \nBNC") -> ("VISA resource name out"=w395:refnum<visa-resource-name>, "error out"=w393:errorcluster)  [unwired: 1 in, 5 out]
        n100 = Build Array(w402, w401, w400, w399) -> (→"appended array":i32[])
        n101 = call-poly "Configure Trigger.vi"("Edge Slope (0: Positive)"="Edge \nSlope", "Input Coupling (0: AC Coupling)"="Input \nCoupling", "error in (no error)"=w393, "Trigger Level (0 V)"="Trigger Level (V)", "Trigger Source (0: Channel 1)"="Trigger Source", "VISA resource name"=w395) -> ("error out"=w392:errorcluster, "VISA resource name out"=w394:refnum<visa-resource-name>)  [unwired: 4 in]
      }
      event Panel Close {
        n102 = event-data() -> ()  [unwired: 1 in, 4 out]
      }
    }
    n103 = local read "Ch1 Vertical Scale"() -> (w21:dbl)
    n104 = local read "Celcius"() -> (w24:dbl)
    n105 = local read "Voltage Level 2"() -> (w30:dbl)
    n106 = local read "Trigger Level (V)"() -> (w29:dbl)
    n107 = local read "Impedance"() -> (w23:i32)
    n108 = case shown="1" w23 {
      tunnel: ["1 MOhm" "50 Ohm"] -> w22
      frame 0, Default {
      }
      frame 1 {
      }
    }
    n109 = Number To Fractional String(number=w24, precision (6)=w20) -> (F-format string=w17:string)  [unwired: 2 in]
    n110 = Number To Fractional String(number=w30, precision (6)=w20) -> (F-format string=w28:string)  [unwired: 2 in]
    n111 = Number To Fractional String(number=w29, precision (6)=w20) -> (F-format string=w27:string)  [unwired: 2 in]
    n112 = Number To Fractional String(number=w21, precision (6)=w20) -> ()  [unwired: 2 in, 1 out]
    n113 = Select(t="Temperature", s="Set Manual Temp?", f=w17) -> (s? t:f=w15:string)
    n114 = Or(x="Close Session", y=w63) -> (x .or. y?=w65:bool)
    n115 = Build Array(w15, w28, w27, w22) -> (w19:string[])
    n116 = case shown="True" "Free Run" {
      tunnel: w44 -> [_ w118]
      tunnel: w43 -> [_ w117]
      tunnel: w42 -> [_ w112]
      tunnel: w32 -> [_ w111]
      tunnel: w31 -> [_ w102]
      tunnel: w19 -> [_ w101]
      tunnel: w18 -> [_ w100]
      frame False {
        w98 = FALSE ("Meas Ind")
        n117 = local write "Meas Ind"(w98) -> ()
        n118 = property on="Meas Ind" class="Bool (strict)"("Blinking"=w98) -> ()  [unwired: 2 in, 2 out]
      }
      frame True {
        w99 = TRUE ("Measurements  ON")
        n119 = property on="Meas Ind" class="Bool (strict)"("Blinking"=w99) -> ()  [unwired: 2 in, 2 out]
        n120 = TDMS Open(9:T1."little-endian" ("byte order (2:little-endian)"), 10:T2."open or create" ("operation (0:open)"), 11:w112) -> (0:w113:errorcluster, 3:w114:refnum<k34>)  [unwired: 4 in]
        n121 = while {
          tunnel: w118 -> [w147]
          tunnel: w117 -> [w146]
          tunnel: w114 -> [w144]
          tunnel: w113 -> [w143]
          tunnel: w111 -> [w142]
          tunnel: [w133] -> w106
          tunnel: [w132] -> w105
          tunnel: w102 -> [w128]
          shift-right: [w126] -> _
          shift-left: dbl[] [] -> [w127]
          i -> [w129]
          stop <- "Stop Button" stop-if-true
          w136 = 4 items=["Peak-Peak", "Maximum", "Mimimum", "Amplitude", "Top", "Base", "Overshoot", "Preshoot", "Average - N Cycles", "Average - Full Screen", "DC RMS - N Cycles", "DC RMS - Full Screen", "AC RMS - N Cycles", "AC RMS - Full Screen (Std Dev)", "Ratio", "Period", "Frequency", "Counter", "+Width", "-Width", "Burst Width", "Duty Cycle", "Rise Time", "Fall Time", "Delay", "Phase", "X minY", "X maxY", "Positive Pulse Count", "Negative Pulse Count", "Raising Edge Count", "Falling Edge Count", "Area - N Cycle", "Area - Full Screen", "Nth Edge Time", "Nth Edge Cross Level Time"] ("Measurement Type (0: Peak-Peak)")
          n122 = call "Read Waveforms (Single).vi"("error in (no error)"=w146, "VISA resource name"=w147) -> ("error out"=w119:errorcluster, "Waveform Data"=w145:waveform(dbl), "VISA resource name out"=w120:refnum<visa-resource-name>)  [unwired: 7 in]
          n123 = Number To Decimal String(number=w129) -> (decimal integer string=w137:string)  [unwired: 1 in]
          n124 = Build Array(w145) -> (w140:waveform(dbl)[])
          n125 = Concatenate Strings("Ch#1, Iteration:" ("group name in (Untitled)"), w137) -> (w131:string)
          n126 = local write "Oscilloscope Waveform"(w140) -> ()
          n127 = Build Array(w131) -> (w141:string[])
          n128 = call-poly "Read Measurement.vi"("VISA resource name"=w120, "Measurement Type (0: Peak-Peak)"=w136, "error in (no error)"=w119) -> ("Result Value"=w121:dbl)  [unwired: 10 in, 2 out]
          n129 = TDMS Write(0:w144, 5:w142, 7:w141, 9:w140, 11:w143) -> (4:w135:refnum<k34>, 15:w134:errorcluster)  [unwired: 1 in, 2 out]
          n130 = Build Array(w121) -> (w130:dbl[])
          n131 = Build Array (concatenate)(w127, w121) -> (w126:dbl[])
          n132 = call <vilib>:"General Histogram.vi"("X"=w126, "max"=0.4, "min"=0.0, "# bins"=256) -> ("Histogram Graph"=w122:T4)  [unwired: 7 in, 4 out]
          n133 = TDMS Write(0:w135, 5:w128, 7:w131, 9:w130, 11:w134) -> (4:w133:refnum<k34>, 15:w132:errorcluster)  [unwired: 1 in, 2 out]
          n134 = local write "XY Graph"(w122) -> ()
          "Frames Recorded" <- w129
        }
        n135 = TDMS Set Properties(5:w101, 7:w100, 8:w105, 10:w102, 11:w106) -> (0:w103:errorcluster, 3:w104:refnum<k34>)  [unwired: 1 in, 2 out]
        n136 = TDMS Close(8:w103, 11:w104) -> ()  [unwired: 2 out]
        n137 = property on="XY Graph" class="XYGraph (strict)"("XScale.NameLbl.Text"="Amplitude" ("X Scale.Unit Label.Text"), "YScale.NameLbl.Text"="Counts" ("Y Scale.Name Label.Text"), "Caption.Text"="Spectrum") -> ()  [unwired: 2 in, 2 out]
        "Meas Ind" <- w99
      }
    }
    n138 = local read "Results Directory"() -> (w25:path)
    n139 = case shown="True" "Settings Button" {
      tunnel: w19 -> [_ w91]
      tunnel: w18 -> [_ w90]
      tunnel: w25 -> [_ w89]
      frame False {
      }
      frame True {
        n140 = TDMS Open(9:T1."little-endian" ("byte order (2:little-endian)"), 10:T2."open or create" ("operation (0:open)"), 11:w89) -> (0:w92:errorcluster, 3:w95:refnum<k34>)  [unwired: 4 in]
        n141 = TDMS Set Properties(5:w91, 7:w90, 8:w92, 11:w95) -> (0:w93:errorcluster, 3:w94:refnum<k34>)  [unwired: 2 in, 2 out]
        n142 = TDMS Close(8:w93, 11:w94) -> ()  [unwired: 2 out]
      }
    }
    n143 = case shown="True" "Load file to display" {
      frame False {
      }
      frame True {
        n144 = call "MARS_SiPM_Data_Analysis.vi"() -> ()  [unwired: 12 in]
      }
    }
  }
  n145 = call "Close.vi"("error in (no error)"=w9, "VISA resource name"=w10) -> ("error out"=w13:errorcluster)  [unwired: 9 out]
  n146 = call <vilib>:"Simple Error Handler.vi"("error in (no error)"=w13) -> ()  [unwired: 1 in, 8 out]
